vi "AlazarGetParameter.vi"(4 "error in (no error)":errorcluster, 5 "Parameter":u32(ring)=268435465 items=["Data Width"=268435465, "Set/Get Async BuffSize"=268435513, "Set/Get Async Buffcount"=268435520, "Get Data Format"=268435522, "Get Samples Per Timestamp Clock"=268435524, "Get Records Captured"=268435525, "Get Async Buffers Pending"=268435536, "Get Async Buffers Pending Full"=268435537, "Get Async Buffers Pending Empty"=268435538, "ECC Mode"=268435528, "Get Aux Input Level"=268435529, "Get Channels Per Board"=268435568, "Pack Mode"=268435570, "Get FPGA Temperature"=268435584], 6 "Channel":u8(ring)=1 items=["A"=1, "B"=2, "C"=4, "D"=8], 7 "Handle":u64) -> (0 "error out":errorcluster, 1 "Return Code":u32, 2 "Value":i32, 3 "Handle":u64)   [LabVIEW 2018]
doc: "Get a device attribute as a signed long value."
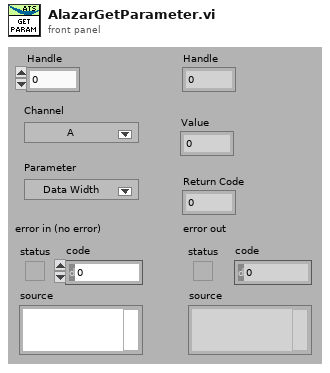
[diagram p1: front panel]
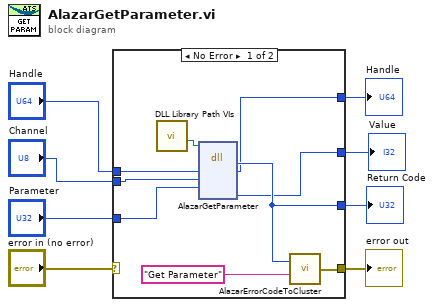
[diagram p0: block diagram]
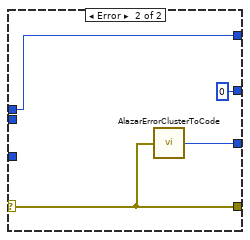
[diagram p2: hidden frame]
diagram:
  n1 = case shown="No Error" "error in (no error)" {
    selector: "error in (no error)" -> [_ w21]
    tunnel: [w14 w21] -> w7
    tunnel: [w16 w20] -> w6
    tunnel: "Handle" -> [w17 w19]
    tunnel: [w13 w19] -> w4
    tunnel: "Channel" -> [w12 _]
    tunnel: "Parameter" -> [w11 _]
    tunnel: [w10 0] -> w1
    frame No Error {
      n2 = call "DLL Library Path VIs.vi"() -> ("Alazar"=w9:path)  [unwired: 9 in, 2 out]
      n3 = dll-call lib="C:/Project/SerialSectOCT - FFT GPU/SerialSectOCT/Labview Software/DLL/ATSApi.dll" fn="AlazarGetParameter"(path in=w9, "handle"=w17, "Channel"=w12, "Parameter"=w11) -> ("return type"=w16:u32, "handle"=w13:u64, "Value"=w10:i32)  [unwired: 5 in, 2 out]
      n4 = call "AlazarErrorCodeToCluster.vi"("Message"="Get Parameter", "Error Code"=w16) -> ("error out"=w14:errorcluster)
    }
    frame Error {
      n5 = call "AlazarErrorClusterToCode.vi"("error in (no error)"=w21) -> ("Error Code"=w20:u32)
    }
  }
  "Handle" <- w4
  "error out" <- w7
  "Return Code" <- w6
  "Value" <- w1
